vi "Write PS Driver.vi"(8 "error in (no error)":errorcluster, 10 "PS Driver.lvlib:PS Driver.lvclass":refnum<class "PS Driver.lvclass">, 11 "PS Control Persistence Actor in":refnum<class "PS Control Persistence Actor.lvclass">) -> (0 "error out":errorcluster, 3 "PS Control Persistence Actor out":refnum<class "PS Control Persistence Actor.lvclass">)   [LabVIEW 2019, in "PS Control Persistence.lvlib" / "PS Control Persistence Actor.lvclass"]
uses:
  PS Control Persistence Actor.lvclass
  PS Driver/PS Driver.lvclass
  PS Driver/PS Driver with Persistence.lvclass
  PS Control Persistence Actor.lvclass/PS Control Persistence Actor.ctl
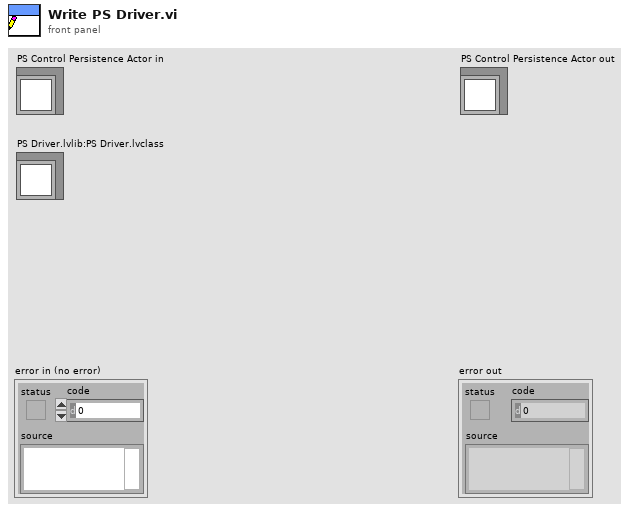
[diagram p1: front panel]
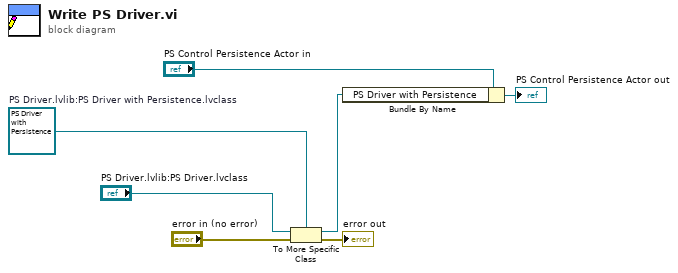
[diagram p0: block diagram]
diagram:
  w4 = refnum<class "PS Driver with Persistence.lvclass"> refnum  # PS Driver.lvlib:PS Driver with Persistence.lvclass
  n1 = To More Specific Class(target class=w4, reference="PS Driver.lvlib:PS Driver.lvclass", error in="error in (no error)") -> (specific class reference=w3:refnum<class "PS Driver with Persistence.lvclass">, error out=→"error out":errorcluster)
  n2 = Bundle By Name(cluster="PS Control Persistence Actor in", "PS Driver with Persistence"=w3) -> (→"PS Control Persistence Actor out":refnum<class "PS Control Persistence Actor.lvclass">)
